vi "MatlabReadTimeTest.vi"() -> ()   [LabVIEW 2017]
panel:
  out "Singles":i32(listbox)
  out "Totals":i32(listbox)
  out "Last array":variant
  out "Read":timestamp
  out "Read size":i32
  out "Convert":timestamp
  out "Generate Matrix":timestamp
  out "Start":timestamp
  in  "MatrixSIze":dbl=1000.0
  in  "Number Of Reads":i32=100
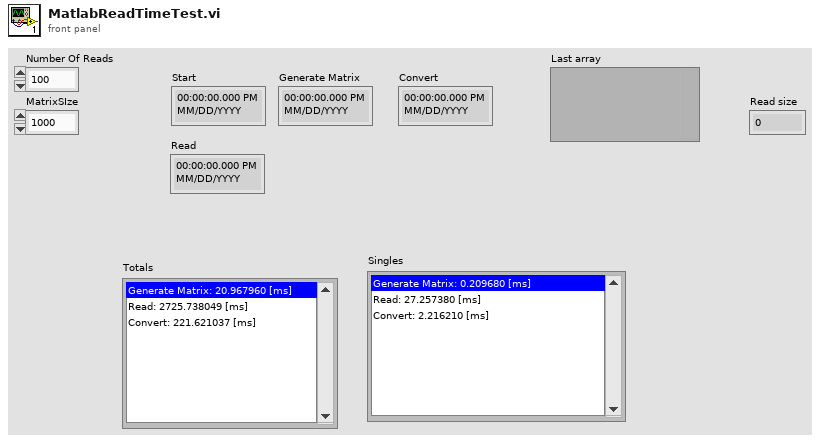
[diagram p1: front panel]
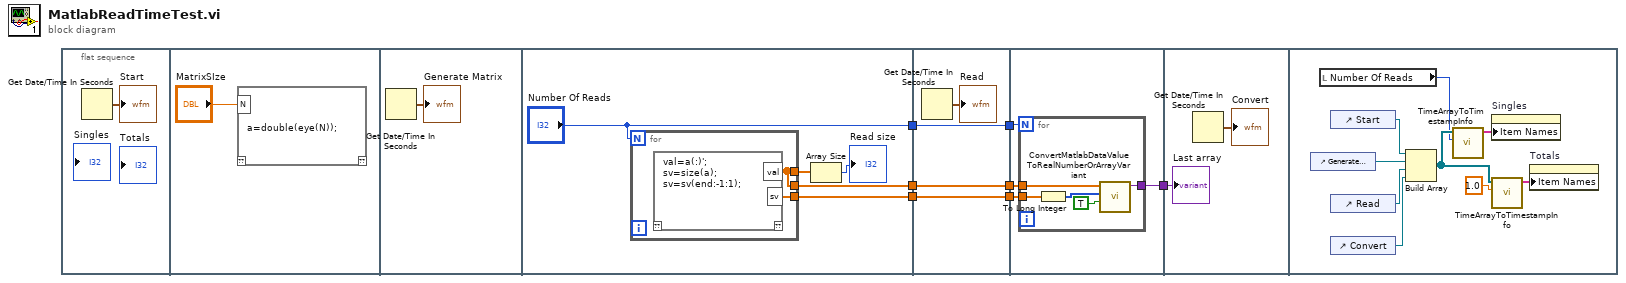
[diagram p0: block diagram]
diagram:
  n1 = flat-sequence {
    tunnel: [w13] -> w7
    tunnel: [w12] -> w5
    tunnel: ["Number Of Reads"] -> w3
    tunnel: w7 -> [w21]
    tunnel: [w21] -> w6
    tunnel: w5 -> [w20]
    tunnel: [w20] -> w4
    tunnel: w3 -> [w19]
    tunnel: [w19] -> w2
    tunnel: w6 -> [w25]
    tunnel: w4 -> [w24]
    tunnel: w2 -> [w23]
    tunnel: [w22] -> w1
    tunnel: w1 -> [w31]
    frame #0 {
      n2 = Get Date/Time In Seconds() -> (seconds since 1Jan1904=→"Start":timestamp)
    }
    frame #1 {
      n3 = script code="a=double(eye(N));"("N"="MatrixSIze") -> ()  [unwired: 1 in, 1 out]
    }
    frame #2 {
      n4 = Get Date/Time In Seconds() -> (seconds since 1Jan1904=→"Generate Matrix":timestamp)
    }
    frame #3 {
      n5 = for {
        N: "Number Of Reads" -> [_]
        tunnel: [w17] -> w15
        tunnel: [w17] -> w13
        tunnel: [w16] -> w12
        n6 = script code="val=a(:)';\nsv=size(a);\nsv=sv(end:-1:1);"() -> ("val"=w17:dbl[], "sv"=w16:dbl[])  [unwired: 1 in, 1 out]
      }
      n7 = Array Size(array=w15) -> (size(s)=→"Read size":i32)
    }
    frame #4 {
      n8 = Get Date/Time In Seconds() -> (seconds since 1Jan1904=→"Read":timestamp)
    }
    frame #5 {
      n9 = for {
        N: w23 -> [_]
        tunnel: w25 -> [w29]
        tunnel: w24 -> [w27]
        tunnel: [w28] -> w22
        n10 = To Long Integer(number=w27) -> (32bit integer=w26:i32[])
        n11 = call "ConvertMatlabDataValueToRealNumberOrArrayVariant.vi"("Has Value"=TRUE, "Sizes"=w26, "Data"=w29) -> ("Reshaped VArray"=w28:variant)  [unwired: 8 in]
      }
    }
    frame #6 {
      n12 = Get Date/Time In Seconds() -> (seconds since 1Jan1904=→"Convert":timestamp)
      "Last array" <- w31
    }
    frame #7 {
      n13 = control-ref of="Generate Matrix"() -> (w40:refnum<vi>)
      n14 = local read "Number Of Reads"() -> (w36:i32)
      n15 = control-ref of="Start"() -> (w41:refnum<vi>)
      n16 = control-ref of="Read"() -> (w39:refnum<vi>)
      n17 = control-ref of="Convert"() -> (w38:refnum<vi>)
      n18 = Build Array(w41, w40, w39, w38) -> (w37:refnum<vi>[])
      n19 = call "TimeArrayToTimestampInfo.vi"("Number of iterations"=w36, "Times array in"=w37) -> ("Array out"=w33:string[])  [unwired: 9 in]
      n20 = property on="Singles" class="LstBox (strict)"("Item Names"=w33) -> ()  [unwired: 2 in, 2 out]
      n21 = call "TimeArrayToTimestampInfo.vi"("Number of iterations"=1.0 ("Times divider"), "Times array in"=w37) -> ("Array out"=w34:string[])  [unwired: 9 in]
      n22 = property on="Totals" class="LstBox (strict)"("Item Names"=w34) -> ()  [unwired: 2 in, 2 out]
    }
  }
